vi "FindEdges.vi"(0 "reference":refnum<class "Graph.lvclass">, 1 "point2D":T1 {"y" format="%.2f"; "x" format="%.2f"}, 2 "GraphicsRef":refnum<class "Graphics.lvclass">, 5 "error in (no error)":errorcluster) -> (14 "reference out":refnum<class "Graph.lvclass">, 15 "Edges":refnum<class "AbstractEdge.lvclass">[](array[class]), 16 "found":bool, 19 "error out":errorcluster)   [LabVIEW 2016, in "Graph.lvclass"]
uses:
  <resource>/Framework/Providers/Open_GDS/UML/Graph_class/Graph.lvclass
  <resource>/Framework/Providers/Open_GDS/UML/General/Point/Point Point2D.ctl
  <resource>/Framework/Providers/Open_GDS/UML/AbstractEdge_class/AbstractEdge.lvclass
  <resource>/Framework/Providers/Open_GDS/UML/Graphics_class/Graphics.lvclass
  <resource>/Framework/Providers/Open_GDS/UML/GeneralPathEdge_class/GeneralPathEdge.lvclass
  C:/Program Files (x86)/National Instruments/LabVIEW 2016/resource/Framework/Providers/Open_GDS/UML/AbstractEdge_class/AbstractEdge.lvclass
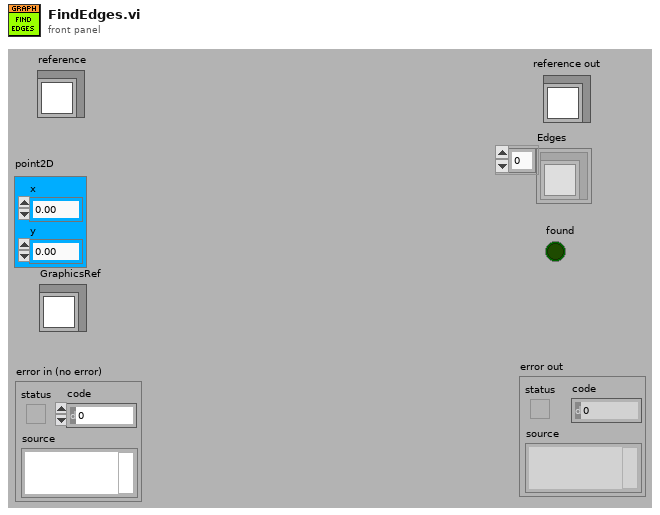
[diagram p1: front panel]
types:
  T1 = typedef "Point Point2D.ctl" = cluster{"x":dbl, "y":dbl}
  T2 = typedef "Graph.lvclass/ObjectAttributes.ctl" = cluster{"nodes":refnum<class "AbstractNode.lvclass">[], "edges":refnum<class "AbstractEdge.lvclass">[], "nodesToBeRemoved":refnum<class "AbstractNode.lvclass">[], "edgesToBeRemoved":refnum<class "AbstractEdge.lvclass">[], "needsLayout":bool, "LayoutNodes":refnum<class "AbstractNode.lvclass">[]}
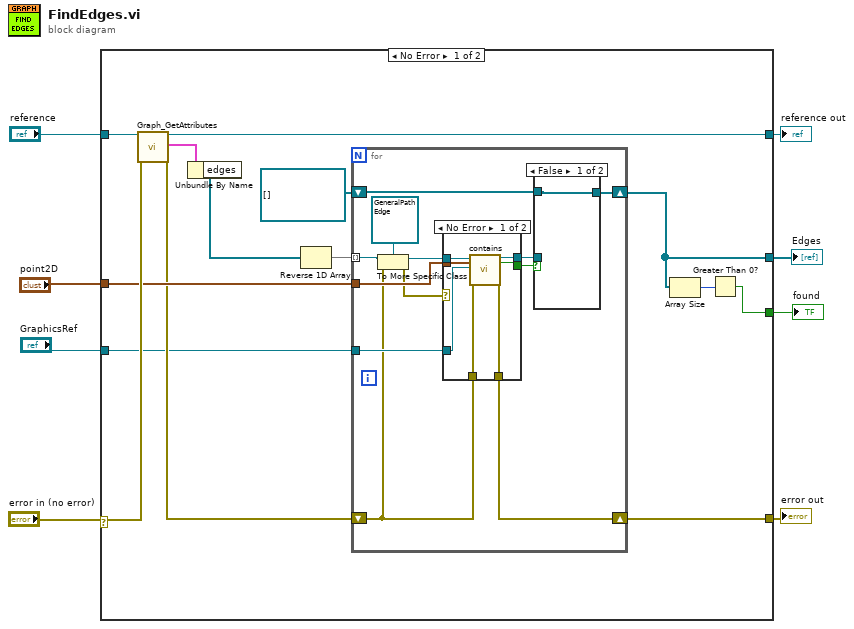
[diagram p0: block diagram]
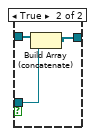
[diagram p3: hidden frame]
diagram:
  n1 = case shown="No Error" "error in (no error)" {
    selector: "error in (no error)" -> [w19 w47]
    tunnel: "reference" -> [w22 w48]
    tunnel: [w21 w47] -> w7
    tunnel: [w20 w48] -> w6
    tunnel: "point2D" -> [w18 _]
    tunnel: [w13 _] -> w3
    tunnel: [w10 _] -> w2
    tunnel: "GraphicsRef" -> [w15 _]
    frame No Error {
      n2 = call <resource>:"Graph_GetAttributes.vi"("reference in"=w22, "error in (no error)"=w19) -> ("reference out"=w20:refnum<class "Graph.lvclass">, "Data"=w9:T2, "error out"=w16:errorcluster)  [unwired: 1 in, 14 out]
      n3 = Unbundle By Name(w9) -> ("edges"=w17:refnum<class "AbstractEdge.lvclass">[])
      n4 = Reverse 1D Array(array=w17) -> (reversed array=w14:refnum<class "AbstractEdge.lvclass">[])
      n5 = for {
        tunnel: w14 -> [w30] mode=indexing
        shift-right: [w34] -> w21
        shift-left: w16 -> [w23]
        tunnel: w18 -> [w33]
        tunnel: w15 -> [w29]
        shift-right: [w25] -> w13
        shift-left: refnum<class "AbstractEdge.lvclass">[] [] -> [w27]
        n6 = To More Specific Class(target class=refnum<class "GeneralPathEdge.lvclass"> refnum ("reference out"), reference=w30, error in=w23) -> (specific class reference=w32:refnum<class "GeneralPathEdge.lvclass">, error out=w24:errorcluster)
        n7 = case shown="No Error" w24 {
          tunnel: w23 -> [w41 w42]
          tunnel: [w40 w42] -> w34
          tunnel: w33 -> [w39 _]
          tunnel: w32 -> [w38 _]
          tunnel: w29 -> [w37 _]
          tunnel: [w36 _] -> w28
          tunnel: [w35 _] -> w26
          frame No Error {
            n8 = call-dynamic "contains.vi"("reference"=w38, "point2D"=w39, "GraphicsRef"=w37, "error in (no error)"=w41) -> ("reference out"=w35:refnum<class "GeneralPathEdge.lvclass">, "contains"=w36:bool, "error out"=w40:errorcluster)  [unwired: 13 in]
          }
          frame Error {
          }
        }
        n9 = case shown="False" w28 {
          tunnel: w27 -> [w43 w46]
          tunnel: w26 -> [_ w45]
          tunnel: [w43 w44] -> w25
          frame False {
          }
          frame True {
            n10 = Build Array (concatenate)(w46, w45) -> (w44:refnum<class "AbstractEdge.lvclass">[])
          }
        }
      }
      n11 = Array Size(array=w13) -> (size(s)=w11:i32)
      n12 = Greater Than 0?(x=w11) -> (x > 0?=w10:bool)
    }
    frame Error {
    }
  }
  "reference out" <- w6
  "error out" <- w7
  "found" <- w2
  "Edges" <- w3
